vi "MF-101 I2C dongle with ADT7420.vi"() -> ()   [LabVIEW 8.6]
uses:
  <libdir>/resource/objmgr/ueidaq.rc
  vi.lib/UeiDaq/UeiDaqConfigureTimingForMessagingIO.vi
  vi.lib/UeiDaq/UeiDaqCreateI2CMasterSession.vi
panel:
  out "temperature (deg F)":dbl
  out "ADT7420 ID":string
  in  "Master:Loopback":i32[](array[ring]) items=["None", "Relay", "FPGA"]
  out "Master Read Data String":string
  out "Master Read Count":i32
  out "Master Channel":i32
  in  "Stop":bool
  in  "Bit Rate":i32(ring) items=["100kBitsPerSecond", "400kBitsPerSecond", "1MBitsPerSecond"]
  in  "TTL Level":i32(ring) items=["3.3V", "5V"]
  in  "Secure Shell?":bool
  out "Device Name":string
  in  "Master Resource":string
  # "I2C Burn-In dongle with ADT7420 temp sensor example"
  # "Relay mode"
  # "dongle\n0-2, 2-0\n1-3, 3-1"
  # "Master Configuration"
  # "Master Specific Configuration"
  # "Device info"
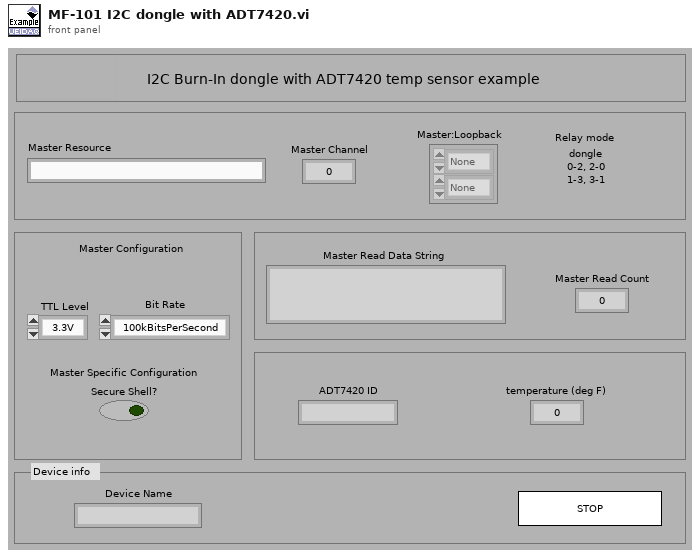
[diagram p1: front panel]
types:
  T1 = cluster{"Command":u32, "Slave Address":i32, "Slave Address Width":u32, "Number Elements to Write":i32, "Number Elements to Read":i32, "Write Data":u8[]}
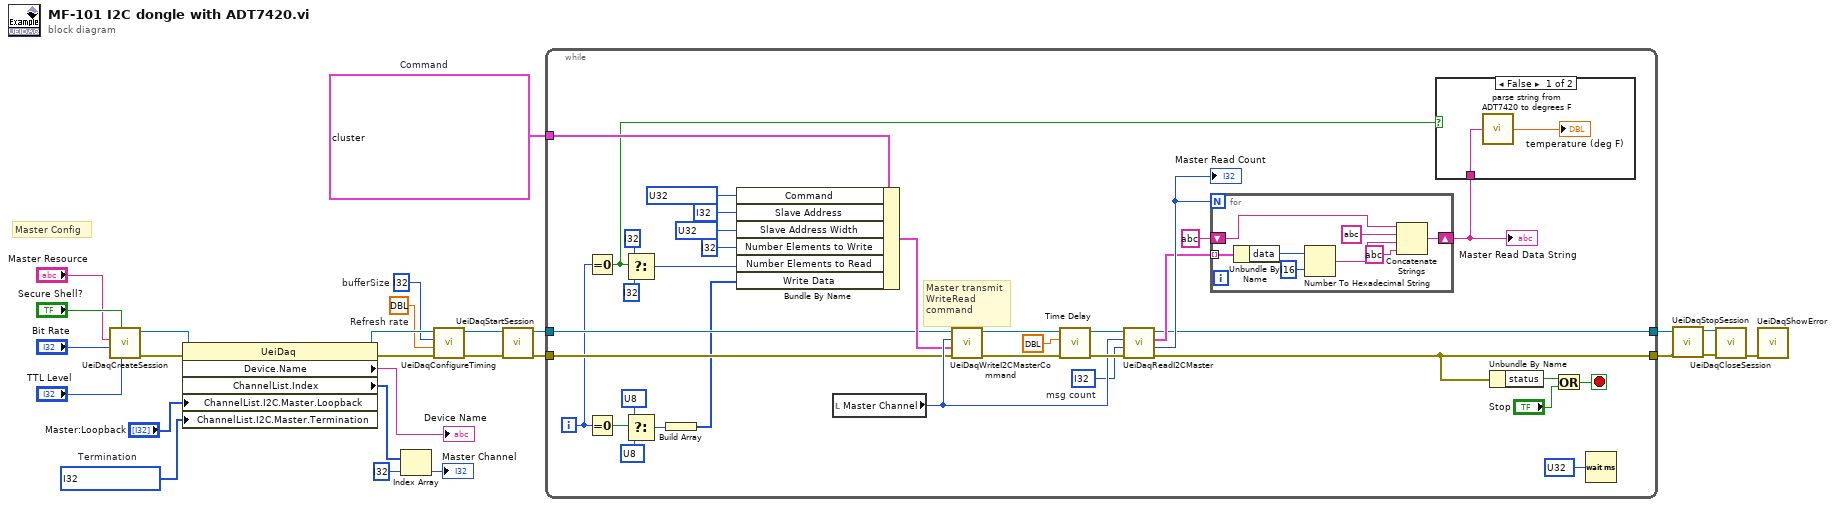
[diagram p0: block diagram]
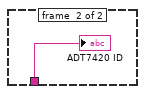
[diagram p2: hidden frame]
diagram:
  w1 = T1 ?  # Command
  w4 = i32[] ? items=["Disabled", "Enabled"]  # Termination
  w6 = dbl ?  # Refresh rate
  w7 = i32 ?  # bufferSize
  # "Master Config"
  n1 = call-poly "UeiDaqCreateSession.vi"("TTL Level"="TTL Level", "Enable Secure Shell"="Secure Shell?", "Bit Rate"="Bit Rate", "Resource"="Master Resource") -> ("error out"=w22:errorcluster, "UeiDaq Refnum Out"=w21:refnum<k20>)  [unwired: 6 in]
  n2 = property class="UeiDaq"(reference=w21, error in=w22, "ChannelList.I2C.Master.Loopback"="Master:Loopback", "ChannelList.I2C.Master.Termination"=w4) -> (reference out=w13:refnum<k20>, error out=w12:errorcluster, "Device.Name"=→"Device Name":string, "ChannelList.Index"=w23:i32[])
  n3 = Index Array(array=w23, index=i32 ?) -> (element=→"Master Channel":i32)
  n4 = call-poly "UeiDaqConfigureTiming.vi"("error in (no error)"=w12, "Refresh rate"=w6, "bufferSize"=w7, "UeiDaq Refnum In"=w13) -> ("error out"=w17:errorcluster, "UeiDaq Refnum Out"=w16:refnum<k20>)  [unwired: 6 in]
  n5 = call "UeiDaqStartSession.vi"("error in (no error)"=w17, "UeiDaq Refnum In"=w16) -> ("error out"=w15:errorcluster, "UeiDaq Refnum Out"=w14:refnum<k20>)  [unwired: 8 in]
  n6 = while {
    tunnel: w15 -> [w44]
    tunnel: w14 -> [w45]
    tunnel: w1 -> [w40]
    tunnel: [w39] -> w3
    tunnel: [w48] -> w2
    i -> [w30]
    stop <- w51 stop-if-true
    w42 = u32 ? items=["7-bit", "10-bit"] ("Slave Address Width")
    w46 = u32 ? items=["Write", "Read", "WriteRead"] ("Command")
    w49 = i32 ?  # msg count
    # "Master transmit\nWriteRead \ncommand"
    n7 = Equal To 0?(x=w30) -> (x = 0?=w28:bool)
    n8 = Equal To 0?(x=w30) -> (x = 0?=w37:bool)
    n9 = Select(t=i32 ? ("Numeric"), s=w28, f=i32 ? ("Numeric")) -> (s? t:f=w29:i32)
    n10 = Select(t=u8 ? ("Numeric"), s=w37, f=u8 ? ("Numeric")) -> (s? t:f=w34:u8)
    n11 = Build Array(w34) -> (w33:u8[])
    n12 = Bundle By Name(cluster=w40, "Command"=w46, "Slave Address"=i32 ?, "Slave Address Width"=w42, "Number Elements to Write"=i32 ?, "Number Elements to Read"=w29, "Write Data"=w33) -> (w47:T1)
    n13 = local read "Master Channel"() -> (w52:i32)
    n14 = call "UeiDaqWriteI2CMasterCommand.vi"("error in (no error)"=w44, "Command"=w47, "Port"=w52, "UeiDaq Refnum In"=w45) -> ("error out"=w56:errorcluster, "UeiDaq Refnum Out"=w58:refnum<k20>)  [unwired: 6 in]
    n15 = call "Time Delay"("error in (no error)"=w56, "Delay Time (s)"=dbl ?) -> ("error out"=w55:errorcluster)  [unwired: 9 in]
    n16 = call "UeiDaqReadI2CMaster.vi"("error in (no error)"=w55, "Message count"=w49, "Port"=w52, "UeiDaq Refnum In"=w58) -> ("error out"=w39:errorcluster, "return count"=w53:i32, "data"=w50:cluster{"stop bit":bool, "data":u8}[], "UeiDaq Refnum Out"=w48:refnum<k20>)  [unwired: 4 in]
    "Master Read Count" <- w53
    n17 = for {
      N: w53 -> [_]
      shift-right: [w70] -> w27
      shift-left: string ? -> [w67]
      tunnel: w50 -> [w65] mode=indexing
      n18 = Unbundle By Name(w65) -> ("data"=w64:u8)
      n19 = Number To Hexadecimal String(1:i16 ? ("width (-)"), 2:w64) -> (0:w71:string)
      n20 = Concatenate Strings(w67, string ? ("string"), w71, string ? ("string")) -> (w70:string)
    }
    "Master Read Data String" <- w27
    n21 = case shown="False" w28 {
      tunnel: w27 -> [w62 w63]
      frame #0 {
        n22 = call "parse string from ADT7420 to degrees F.vi"("Master Read Data String"=w62) -> ("temperature (deg F)"=→"temperature (deg F)":dbl)
      }
      frame #1 {
        "ADT7420 ID" <- w63
      }
    }
    n23 = Unbundle By Name(w39) -> ("status"=w38:bool)
    n24 = Or(x=w38, y="Stop") -> (x .or. y?=w51:bool)
    n25 = Wait (ms)(milliseconds to wait=u32 ?) -> ()  [unwired: 1 out]
  }
  n26 = call "UeiDaqStopSession.vi"("error in (no error)"=w3, "UeiDaq Refnum In"=w2) -> ("error out"=w9:errorcluster, "UeiDaq Refnum Out"=w10:refnum<k20>)  [unwired: 8 in]
  n27 = call "UeiDaqCloseSession.vi"("error in (no error)"=w9, "UeiDaq Refnum In"=w10) -> ("error out"=w26:errorcluster)  [unwired: 1 in, 8 out]
  n28 = call "UeiDaqShowError.vi"("error in (no error)"=w26) -> ()  [unwired: 2 in, 9 out]
